vi "JL Create LED Names_HE.vi"(0 "Expected LEDs":T1={"SSD"="", "Cycle Selection"=enum."Cycle 0", "Bar Selection"=enum."Bar 1", "Temp Setting"=enum."No Heat", "Dryness Level"=enum."Damp", "Time Setting"=enum."Default Time 1", "Dryer Status"=enum."Status 6", "Start/Pause"=FALSE, "Pause"=FALSE, "Control Lock"=FALSE, "Sensing"=FALSE, "Clean Filter"=FALSE, "My Cycle"=FALSE, "Delay Dry"=FALSE, "Volume"=FALSE, "Damp Alert"=FALSE, "Ext Tumble"=FALSE, "Decrement"=FALSE, "Increment"=FALSE, "eDry"=FALSE, "Extra Status"=FALSE}, 11 "Error In":errorcluster) -> (4 "Array of LED Names":string[](array[string]), 15 "Error Out":errorcluster)   [LabVIEW 2016]
uses:
  type defs/JL Display.ctl
  type defs/Cycle Selection Enum.ctl
  type defs/Bar Enum.ctl
  type defs/Temp Setting Enum.ctl
  type defs/Dryness Enum.ctl
  type defs/Time Enum.ctl
  type defs/Status Enum.ctl
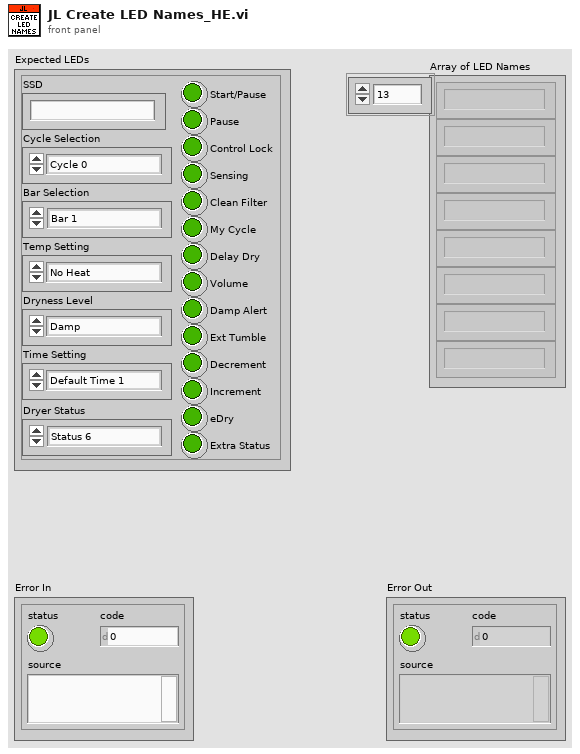
[diagram p1: front panel]
types:
  T1 = typedef "JL Display.ctl" = cluster{"SSD":string, "Cycle Selection":T2, "Bar Selection":T3, "Temp Setting":T4, "Dryness Level":T5, "Time Setting":T6, "Dryer Status":T7, "Start/Pause":bool, "Pause":bool, "Control Lock":bool, "Sensing":bool, "Clean Filter":bool, "My Cycle":bool, "Delay Dry":bool, "Volume":bool, "Damp Alert":bool, "Ext Tumble":bool, "Decrement":bool, "Increment":bool, "eDry":bool, "Extra Status":bool}
  T2 = typedef "Cycle Selection Enum.ctl" = enum16{"Cycle 0", "Cycle 1", "Cycle 2", "Cycle 3", "Cycle 4", "Cycle 5", "Cycle 6", "Cycle 7", "Cycle 8", "Cycle 9", "Cycle 10", "Cycle 11", "Cycle 12", "Cycle 13", "Off", "*Invalid"}
  T3 = typedef "Bar Enum.ctl" = enum16{"Bar 1", "Bar 2", "Bar 3", "Bar 4", "Bar 5", "Off", "*Incorrect*"}
  T4 = typedef "Temp Setting Enum.ctl" = enum16{"Off", "No Heat", "Extra Low", "Low", "Medium", "High", "*Incorrect*"}
  T5 = typedef "Dryness Enum.ctl" = enum16{"Off", "Damp", "Less Dry", "Dry", "More Dry", "Extra Dry", "*Incorrect*"}
  T6 = typedef "Time Enum.ctl" = enum16{"Off", "Default Time 1", "Default Time 2", "Default Time 3", "Default Time 4", "Default Time 5", "*Incorrect*"}
  T7 = typedef "Status Enum.ctl" = enum16{"Status 1", "Status 2", "Status 3", "Status 4", "Status 5", "Status 6", "Off", "*Incorrect*"}
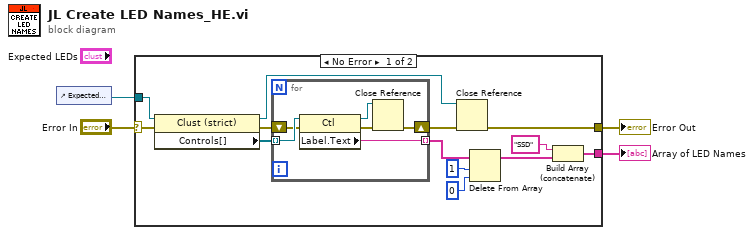
[diagram p0: block diagram]
diagram:
  n1 = control-ref of="Expected LEDs"() -> (w1:refnum<vi>)
  n2 = case shown="No Error" "Error In" {
    selector: "Error In" -> [w8 w24]
    tunnel: w1 -> [w17 _]
    tunnel: [w12 w24] -> w4
    tunnel: [w9 _] -> w3
    frame No Error {
      n3 = property class="Clust (strict)"(reference=w17, error in=w8) -> (reference out=w13:refnum<vi>, error out=w15:errorcluster, "Controls[]"=w16:refnum<vi>[])
      n4 = for {
        tunnel: w16 -> [w23] mode=indexing
        shift-right: [w19] -> w14
        shift-left: w15 -> [w22]
        tunnel: [w18] -> w7 mode=indexing
        n5 = property class="Ctl"(reference=w23, error in=w22) -> (reference out=w21:refnum<vi>, error out=w20:errorcluster, "Label.Text"=w18:string)
        n6 = Close Reference(reference=w21, error in (no error)=w20) -> (error out=w19:errorcluster)
      }
      n7 = Close Reference(reference=w13, error in (no error)=w14) -> (error out=w12:errorcluster)
      n8 = Delete From Array(array=w7, length=1, index=0) -> (array with subset deleted=w6:string[])  [unwired: 1 out]
      n9 = Build Array (concatenate)("SSD", w6) -> (w9:string[])
    }
    frame Error {
    }
  }
  "Error Out" <- w4
  "Array of LED Names" <- w3
